vi "teste-motor-3.vi"() -> ()   [LabVIEW 2014]
doc: "André Romero - 2017\nandretec@ifsc.usp.br"
panel:
  out "Numeric 2":i32
  out "x-y":dbl
  out "GetPOS ABS 2":dbl=2.699072994402985
  out "GetPOS ABS 1":dbl=2.699072994402985
  in  "Ciclos":i32=100
  out "Numeric":i32
  out "GetPOS X":dbl=10.0 format="%#_6e"
  in  "GO Move":bool
  out "Motor 2":bool
  out "Motor 1":bool
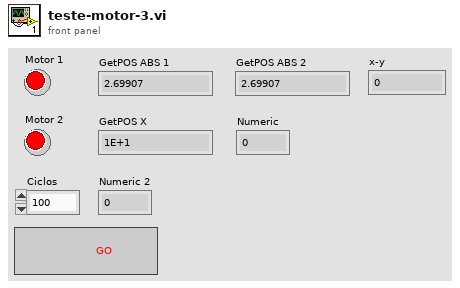
[diagram p1: front panel]
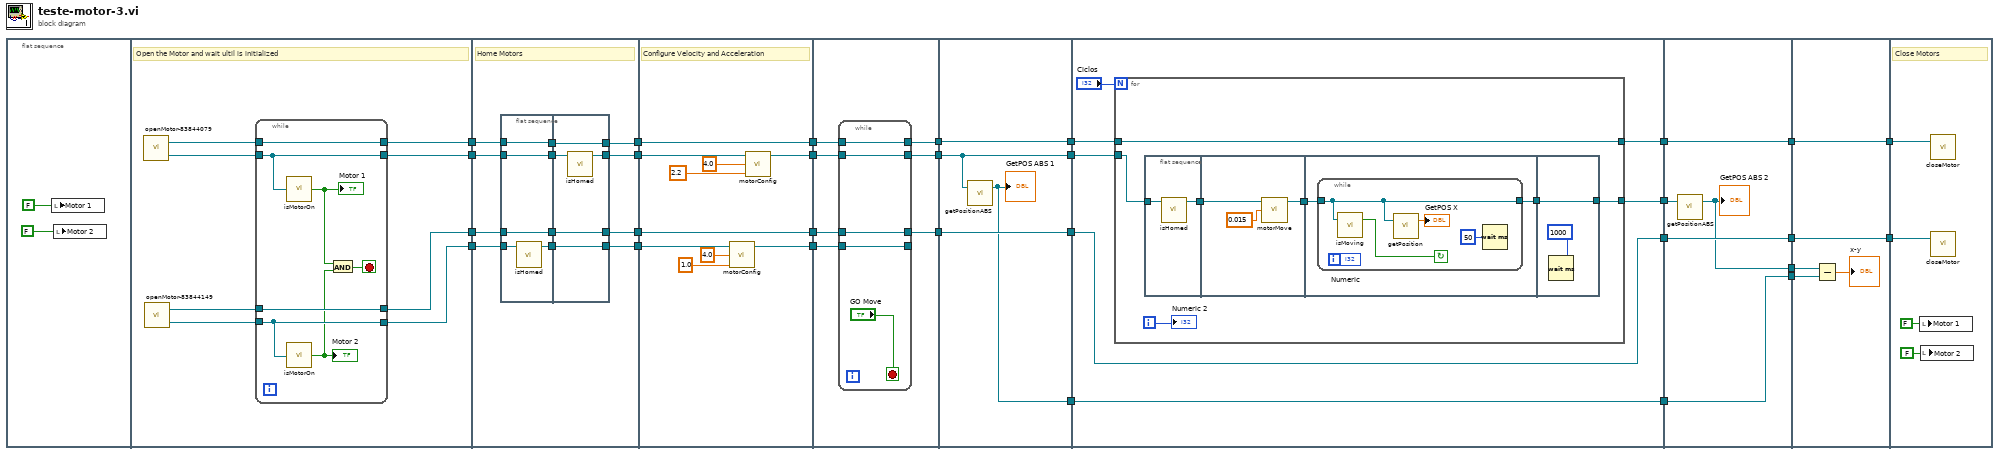
[diagram p0: block diagram]
diagram:
  n1 = flat-sequence {
    tunnel: [w37] -> w29
    tunnel: [w36] -> w28
    tunnel: [w33] -> w27
    tunnel: [w32] -> w26
    tunnel: w29 -> [w54]
    tunnel: w28 -> [w53]
    tunnel: [w56] -> w23
    tunnel: w27 -> [w55]
    tunnel: [w57] -> w21
    tunnel: w26 -> [w58]
    tunnel: [w48] -> w25
    tunnel: [w47] -> w19
    tunnel: w25 -> [w77]
    tunnel: [w77] -> w24
    tunnel: w23 -> [w78]
    tunnel: [w78] -> w22
    tunnel: w21 -> [w73]
    tunnel: [w69] -> w20
    tunnel: w19 -> [w76]
    tunnel: [w70] -> w18
    tunnel: w24 -> [w85]
    tunnel: [w84] -> w11
    tunnel: w22 -> [w82]
    tunnel: w20 -> [w81]
    tunnel: w18 -> [w83]
    tunnel: [w80] -> w9
    tunnel: [w79] -> w7
    tunnel: w11 -> [w94]
    tunnel: [w94] -> w10
    tunnel: w9 -> [w92]
    tunnel: [w92] -> w8
    tunnel: w7 -> [w93]
    tunnel: [w93] -> w6
    tunnel: [w91] -> w3
    tunnel: w10 -> [w100]
    tunnel: [w99] -> w15
    tunnel: w8 -> [w98]
    tunnel: [w97] -> w13
    tunnel: w6 -> [w97]
    tunnel: [w96] -> w5
    tunnel: w3 -> [w95]
    tunnel: [w95] -> w2
    tunnel: w15 -> [w127]
    tunnel: [w127] -> w14
    tunnel: w13 -> [w126]
    tunnel: [w126] -> w12
    tunnel: w5 -> [w125]
    tunnel: [w124] -> w4
    tunnel: w2 -> [w123]
    tunnel: [w123] -> w1
    tunnel: w14 -> [w132]
    tunnel: [w132] -> w17
    tunnel: w12 -> [w131]
    tunnel: [w131] -> w16
    tunnel: w4 -> [w130]
    tunnel: w1 -> [w129]
    tunnel: w17 -> [w136]
    tunnel: w16 -> [w133]
    frame #0 {
      n2 = local write "Motor 1"(FALSE ("isConnected")) -> ()
      n3 = local write "Motor 2"(FALSE ("isConnected 2")) -> ()
    }
    frame #1 {
      # "Open the Motor and wait ultil is initialized"
      n4 = call "openMotor-83844079.vi"() -> ("Device"=w38:refnum<k24>, ".NET Refnum out"=w39:refnum<k24>)  [unwired: 2 in]
      n5 = call "openMotor-83844149.vi"() -> ("Device"=w35:refnum<k24>, ".NET Refnum out"=w34:refnum<k24>)  [unwired: 2 in]
      n6 = while {
        tunnel: w39 -> [w46]
        tunnel: [w46] -> w37
        tunnel: w38 -> [w45]
        tunnel: [w45] -> w36
        tunnel: w35 -> [w43]
        tunnel: [w44] -> w33
        tunnel: w34 -> [w44]
        tunnel: [w43] -> w32
        stop <- w40 stop-if-true
        n7 = call "isMotorOn.vi"("Device"=w45) -> ("isConnected"=w41:bool)
        "Motor 1" <- w41
        n8 = call "isMotorOn.vi"("Device"=w43) -> ("isConnected"=w42:bool)
        "Motor 2" <- w42
        n9 = And(x=w41, y=w42) -> (x .and. y?=w40:bool)
      }
    }
    frame #2 {
      # "Home Motors"
      n10 = flat-sequence {
        tunnel: w58 -> [w63]
        tunnel: w55 -> [w61]
        tunnel: w54 -> [w60]
        tunnel: w53 -> [w59]
        tunnel: [w62] -> w52
        tunnel: [w61] -> w51
        tunnel: [w60] -> w50
        tunnel: [w59] -> w49
        tunnel: [w64] -> w47
        tunnel: [w66] -> w48
        tunnel: [w67] -> w56
        tunnel: [w68] -> w57
        tunnel: w52 -> [w68]
        tunnel: w51 -> [w67]
        tunnel: w50 -> [w66]
        tunnel: w49 -> [w65]
        frame #0 {
          n11 = call "isHomed.vi"("Device in"=w63) -> ("Device out"=w62:refnum<k24>)  [unwired: 4 in]
        }
        frame #1 {
          n12 = call "isHomed.vi"("Device in"=w65) -> ("Device out"=w64:refnum<k24>)  [unwired: 4 in]
        }
      }
    }
    frame #3 {
      # "Configure Velocity and Acceleration"
      n13 = call "motorConfig.vi"("Velocity"=1.0 ("MaxVelocity"), "Acceleration"=4.0, "Device in"=w73) -> ("Device out"=w69:refnum<k24>)  [unwired: 2 in]
      n14 = call "motorConfig.vi"("Velocity"=2.2 ("MaxVelocity"), "Acceleration"=4.0, "Device in"=w76) -> ("Device out"=w70:refnum<k24>)  [unwired: 2 in]
    }
    frame #4 {
      n15 = while {
        tunnel: [w89] -> w84
        tunnel: w85 -> [w89]
        tunnel: [w88] -> w80
        tunnel: w83 -> [w88]
        tunnel: w82 -> [w86]
        tunnel: [w87] -> _
        tunnel: w81 -> [w87]
        tunnel: [w86] -> w79
        stop <- "GO Move" stop-if-true
      }
    }
    frame #5 {
      n16 = call "getPositionABS.vi"("Device"=w92) -> ("Device out"=w91:refnum<k24>)  [unwired: 1 in, 1 out]
      "GetPOS ABS 1" <- w91
    }
    frame #6 {
      n17 = for {
        N: "Ciclos" -> [_]
        tunnel: w100 -> [w108]
        tunnel: [w108] -> w99
        tunnel: w98 -> [w106]
        tunnel: [w104] -> w96
        i -> [w103]
        n18 = flat-sequence {
          tunnel: [w110] -> w107
          tunnel: w106 -> [w109]
          tunnel: w107 -> [w112]
          tunnel: [w111] -> w105
          tunnel: w105 -> [w115]
          tunnel: [w114] -> w102
          tunnel: [w122] -> w104
          tunnel: w102 -> [w122]
          frame #0 {
            n19 = call "isHomed.vi"("Device in"=w109) -> ("Device out"=w110:refnum<k24>)  [unwired: 4 in]
          }
          frame #1 {
            n20 = call "motorMove.vi"("position"=0.015, "Device in"=w112) -> ("Device out"=w111:refnum<k24>)  [unwired: 3 in]
          }
          frame #2 {
            n21 = while {
              tunnel: w115 -> [w120]
              tunnel: [w120] -> w114
              i -> [w117]
              stop <- w119 continue-if-true
              n22 = call "isMoving.vi"("Device in"=w120) -> ("IsMoving"=w119:bool)  [unwired: 1 in, 1 out]
              n23 = call "getPosition.vi"("Device"=w120) -> ("GetPOS"=→"GetPOS X":dbl)  [unwired: 2 in]
              n24 = Wait (ms)(milliseconds to wait=u32 50) -> ()  [unwired: 1 out]
              "Numeric" <- w117
            }
          }
          frame #3 {
            n25 = Wait (ms)(milliseconds to wait=u32 1000) -> ()  [unwired: 1 out]
          }
        }
        "Numeric 2" <- w103
      }
    }
    frame #7 {
      n26 = call "getPositionABS.vi"("Device"=w125) -> ("Device out"=w124:refnum<k24>)  [unwired: 1 in, 1 out]
      "GetPOS ABS 2" <- w124
    }
    frame #8 {
      n27 = Subtract(x=w130, y=w129) -> (x-y=→"x-y":dbl)
    }
    frame #9 {
      # "Close Motors"
      n28 = local write "Motor 1"(FALSE ("Motor 1")) -> ()
      n29 = local write "Motor 2"(FALSE ("Motor 2")) -> ()
      n30 = call "closeMotor.vi"(".NET Refnum in"=w136) -> ()  [unwired: 2 in]
      n31 = call "closeMotor.vi"(".NET Refnum in"=w133) -> ()  [unwired: 2 in]
    }
  }
